vi "Set Log File.vi"(8 "error in (no error)":errorcluster, 10 "Log File":path, 11 "CLILogger in":refnum<class "CLILogger.lvclass">) -> (0 "error out":errorcluster, 3 "CLILogger out":refnum<class "CLILogger.lvclass">)   [LabVIEW 2020, in "GPackTools.lvlib" / "CLILogger.lvclass"]
uses:
  CLILogger.lvclass
  CLILogger.lvclass/CLILogger.ctl
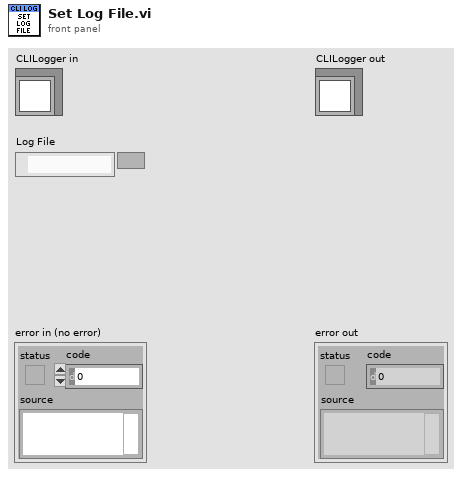
[diagram p1: front panel]
types:
  T1 = enum16{"open", "replace", "create", "open or create", "replace or create", "replace or create with confirmation"}
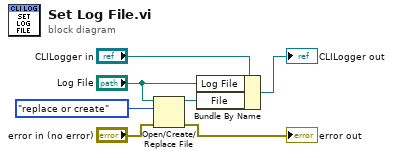
[diagram p0: block diagram]
diagram:
  n1 = Open/Create/Replace File(file path (use dialog)="Log File", error in="error in (no error)", operation (0:open)=T1."replace or create") -> (refnum out=w1:refnum<file>, error out=→"error out":errorcluster)  [unwired: 3 in, 1 out]
  n2 = Bundle By Name(cluster="CLILogger in", "Log File"="Log File", "File"=w1) -> (→"CLILogger out":refnum<class "CLILogger.lvclass">)
